vi "PRIVATE.ProcCases.vi"(0 "i ref in":refnum<vi>, 1 "selector":string, 2 "Data":T1, 3 "call cluster":T2={"Object"="", "Selector"="", "CallType"=enum."synchronous", "Async Object"="", "Async Selector"="", "Data Descriptor"="", "Data"=[], "Error #"=0, "Expire"=0}, 5 "error in (no error)":errorcluster) -> (14 "i ref out":refnum<vi>, 17 "answer cluster":T2={"Object"="", "Selector"="", "CallType"=enum."synchronous", "Async Object"="", "Async Selector"="", "Data Descriptor"="", "Data"=[], "Error #"=0, "Expire"=0}, 19 "error out":errorcluster)   [LabVIEW 2014, in "IMAQDevice.lvlib"]
doc: "This method is called by a process from within the default case in the event loop. The methods of a class that are linked to events will be called from THIS method. Add your code here."
uses:
  IMAQDevice.lvlib
  CSCore/CSSystem/CoreLib/CoreLib.lvlib
  CSCore/BaseProcess/BaseProcess.lvlib
  CSCore/CSSystem/CoreLib/CoreLib.string 2 byte array.vi
  CSCore/CSSystem/CoreLib/CoreLib.byte array 2 double.vi
  CSCore/CSSystem/CoreLib/CoreLib.double 2 byte array.vi
  CSCore/CSSystem/CoreDefs/CoreDefs.call_type.ctl
  CSCore/CSSystem/CoreDefs/CoreDefs.rawDataType.ctl
  CSCore/BaseProcess/BaseProcess.descriptor string definition.ctl
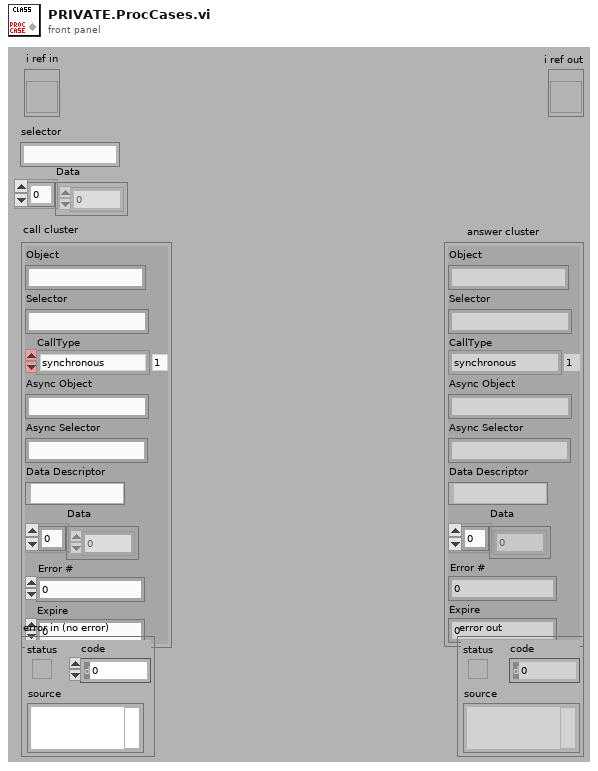
[diagram p1: front panel]
types:
  T1 = typedef "CoreDefs.rawDataType.ctl" = i8[]
  T2 = typedef "CoreDefs.call_type.ctl" = cluster{"Object":string, "Selector":string, "CallType":enum16{"simple", "synchronous", "asynchronous"}, "Async Object":string, "Async Selector":string, "Data Descriptor":T3, "Data":T1, "Error #":i32, "Expire":u32}
  T3 = typedef "BaseProcess.lvlib/BaseProcess.descriptor string definition.ctl" = string
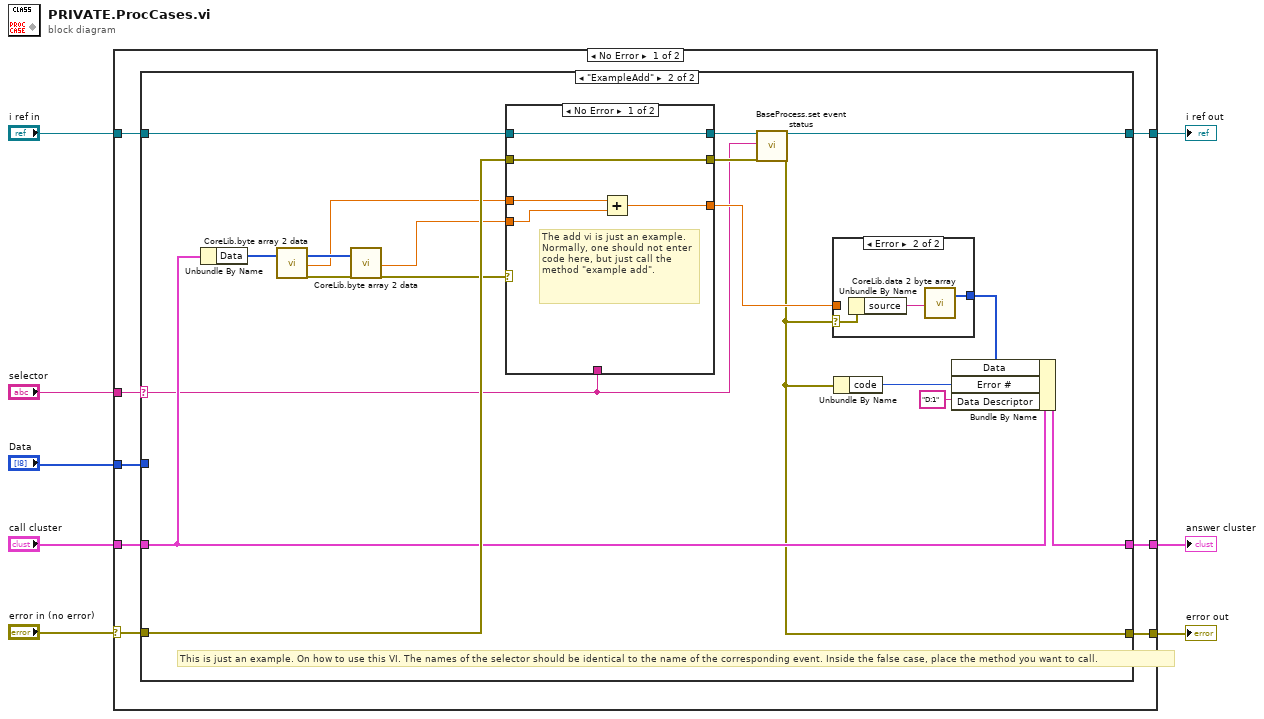
[diagram p0: block diagram]
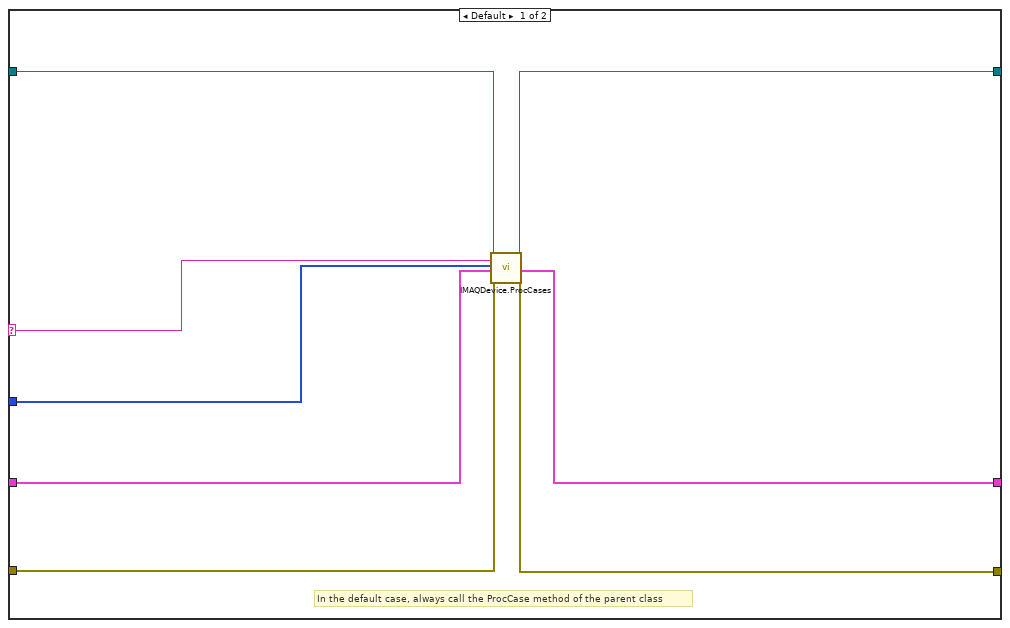
[diagram p2: hidden frame]
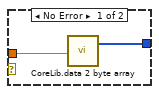
[diagram p3: hidden frame]
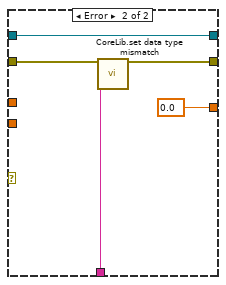
[diagram p4: hidden frame]
diagram:
  n1 = case shown="No Error" "error in (no error)" {
    selector: "error in (no error)" -> [w9 w59]
    tunnel: "selector" -> [w16 _]
    tunnel: [w15 w60] -> w7
    tunnel: "Data" -> [w14 _]
    tunnel: "call cluster" -> [w13 w60]
    tunnel: "i ref in" -> [w12 w61]
    tunnel: [w11 w61] -> w3
    tunnel: [w10 w59] -> w2
    frame No Error {
      n2 = case shown="\"ExampleAdd\"" w16 {
        selector: w16 -> [w19 w33]
        tunnel: w14 -> [w17 _]
        tunnel: w12 -> [w18 w43]
        tunnel: [w24 w32] -> w11
        tunnel: w13 -> [w20 w39]
        tunnel: [w21 w38] -> w15
        tunnel: w9 -> [w23 w42]
        tunnel: [w22 w34] -> w10
        frame Default {
          # "In the default case, always call the ProcCase method of the parent class"
          n3 = call "IMAQDevice.ProcCases.vi"("i ref in"=w18, "selector"=w19, "Data"=w17, "call cluster"=w20, "error in (no error)"=w23) -> ("i ref out"=w24:refnum<vi>, "answer cluster"=w21:T2, "error out"=w22:errorcluster)  [unwired: 12 in]
        }
        frame "ExampleAdd" {
          # "This is just an example. On how to use this VI. The names of the selector should be identical to the name of the corresponding event. Inside the false case, place the method you want to call."
          n4 = Unbundle By Name(w39) -> ("Data"=w30:T1)
          n5 = call-poly "CoreLib.byte array 2 data.vi"("byteArray"=w30) -> ("byteArray out"=w28:T1, "d64"=w26:dbl, "error out"=w29:errorcluster)  [unwired: 16 in]
          n6 = call-poly "CoreLib.byte array 2 data.vi"("byteArray"=w28, "error in (no error)"=w29) -> ("d64"=w25:dbl, "error out"=w27:errorcluster)  [unwired: 15 in, 1 out]
          n7 = case shown="No Error" w27 {
            tunnel: [w50 w58] -> w36
            tunnel: w43 -> [w50 w58]
            tunnel: w42 -> [w51 w57]
            tunnel: [w51 w56] -> w35
            tunnel: w25 -> [w53 _]
            tunnel: [w52 0.0] -> w41
            tunnel: w33 -> [_ w54]
            tunnel: w26 -> [w49 _]
            frame No Error {
              # "The add vi is just an example. Normally, one should not enter code here, but just call the method \"example add\"."
              n8 = Add(x=w49, y=w53) -> (x+y=w52:dbl)
            }
            frame Error {
              n9 = call "CoreLib.set data type mismatch.vi"("error in (no error)"=w57, "error source"=w54) -> ("error out"=w56:errorcluster)  [unwired: 17 in]
            }
          }
          n10 = call "BaseProcess.set event status.vi"("i ref in"=w36, "EventStatus"=w33, "error in (no error)"=w35) -> ("i ref out"=w32:refnum<vi>, "error out"=w34:errorcluster)  [unwired: 14 in, 1 out]
          n11 = case shown="Error" w34 {
            selector: w34 -> [_ w48]
            tunnel: [w44 w47] -> w37
            tunnel: w41 -> [w45 _]
            frame No Error {
              n12 = call-poly "CoreLib.data 2 byte array.vi"("f64"=w45) -> ("byteArray out"=w44:T1)  [unwired: 18 in]
            }
            frame Error {
              n13 = Unbundle By Name(w48) -> ("source"=w46:string)
              n14 = call-poly "CoreLib.data 2 byte array.vi"("string"=w46) -> ("byteArray out"=w47:T1)  [unwired: 18 in]
            }
          }
          n15 = Unbundle By Name(w34) -> ("code"=w40:i32)
          n16 = Bundle By Name(cluster=w39, "Data"=w37, "Error #"=w40, "Data Descriptor"="D:1") -> (w38:T2)
        }
      }
    }
    frame Error {
    }
  }
  "answer cluster" <- w7
  "i ref out" <- w3
  "error out" <- w2
